vi "Main.vi"   [LabVIEW 2017, in "PrototypePatternDemo.lvclass"]
uses:
  PrototypePatternDemo.lvclass
  ConsoleOut/Print Options.ctl
  BundledShapeCache Class/BundledShapeCache.lvclass
  Shape Class/pShape.lvclass
  Circle Class/pCircle.lvclass
  Rectangle Class/pRectangle.lvclass
  C:/Users/fflores/Documents/LabVIEW-Open-Projects/LabIVEW OOP Design Patterns/Prototype Pattern/Shape Class/pShape.lvclass
types:
  T1 = typedef "Print Options.ctl" = enum16{"Create", "Get Reference", "Print", "Print Header", "Close"}
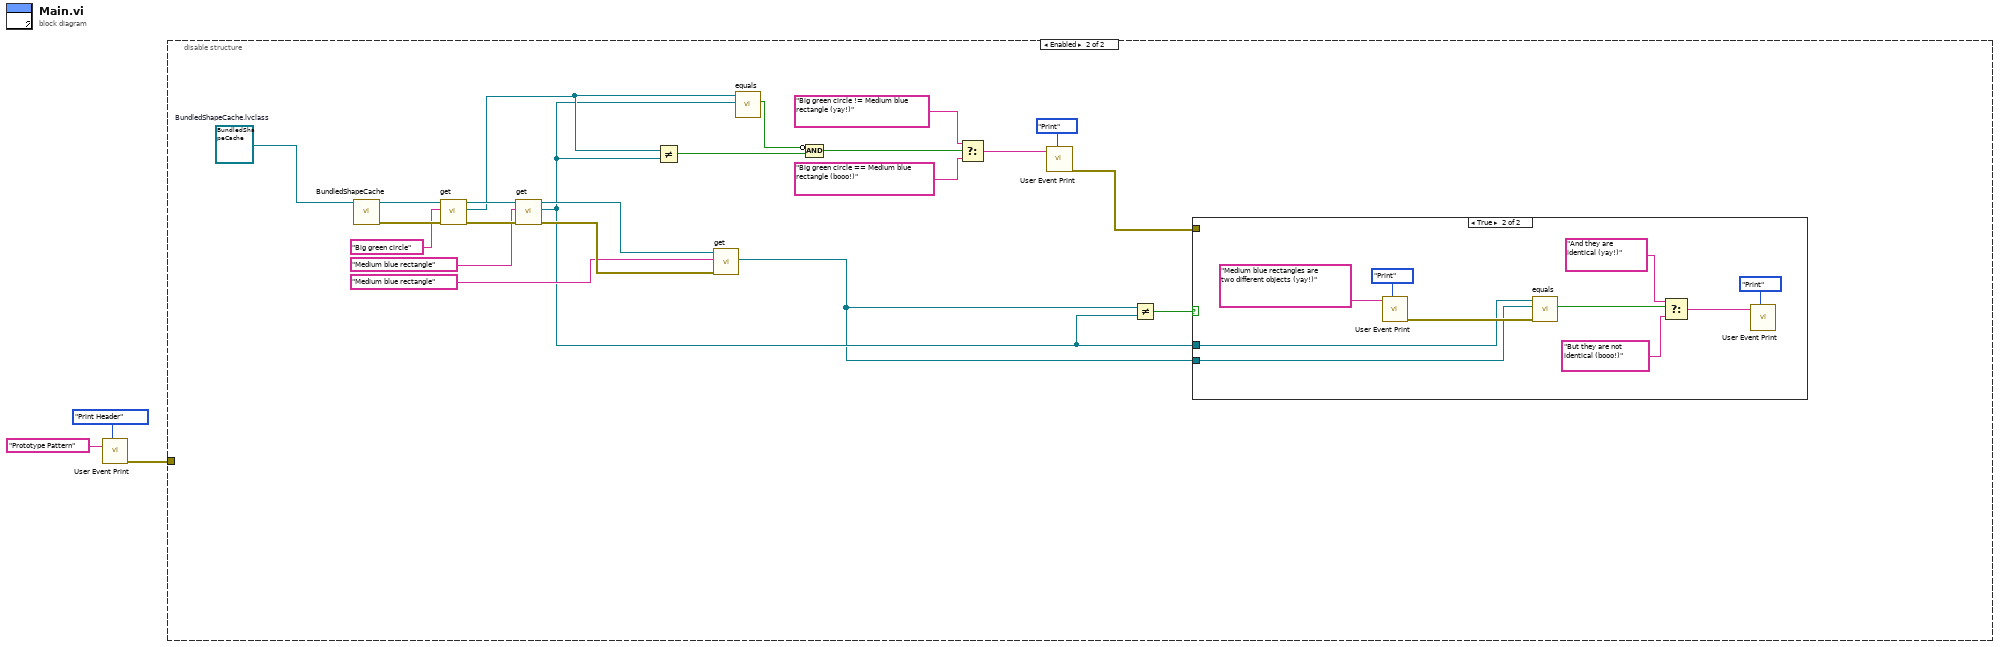
[diagram p0: block diagram]
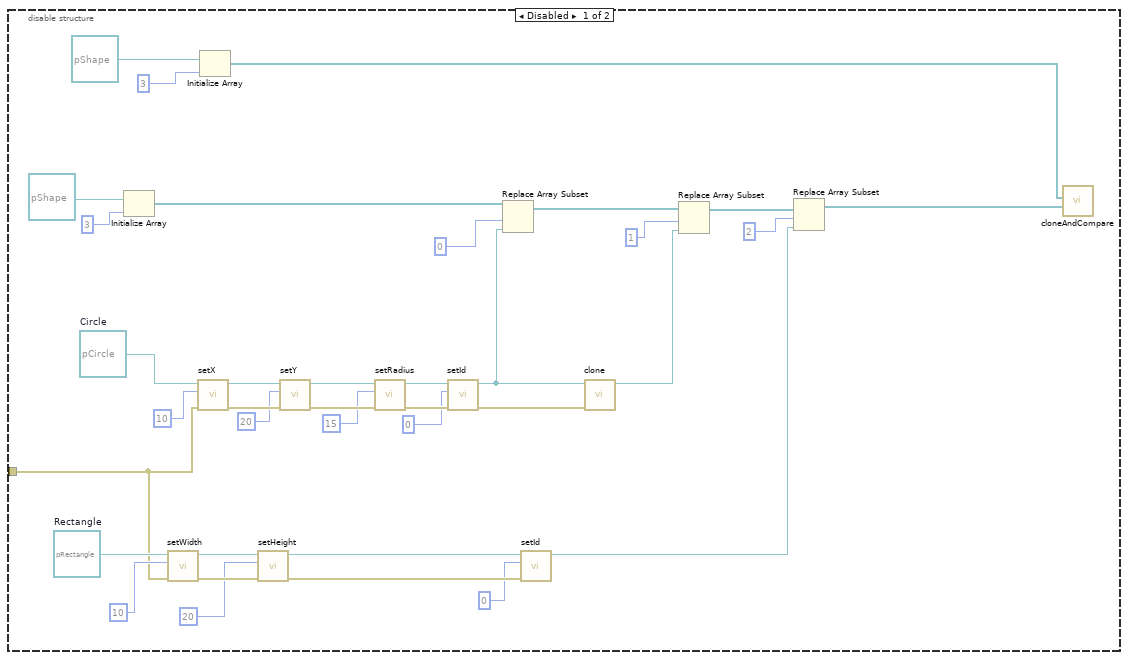
[diagram p2: hidden frame]
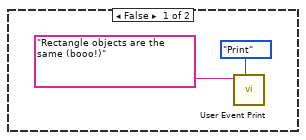
[diagram p3: hidden frame]
diagram:
  n1 = call "User Event Print.vi"("Options"=Print_Options."Print Header", "String to Print"="Prototype Pattern") -> ("error out"=w3:errorcluster)  [unwired: 8 in, 1 out]
  n2 = disable-structure shown="Enabled" {
    disable-tunnel: w3 -> [w12 _]
    frame Disabled {
      w28 = refnum<class "pRectangle.lvclass"> refnum  # Rectangle
      w35 = refnum<class "pCircle.lvclass"> refnum  # Circle
      n3 = Initialize Array(refnum<class "pShape.lvclass"> refnum ("pShape.lvclass"), 3 ("dimension size")) -> (w23:refnum<class "pShape.lvclass">[])
      n4 = call "setWidth.vi"("error in (no error)"=w12, "width"=10, "pRectangle in"=w28) -> ("error out"=w29:errorcluster, "pRectangle out"=w30:refnum<class "pRectangle.lvclass">)  [unwired: 7 in]
      n5 = call "setX.vi"("error in (no error)"=w12, "x"=10, "pCircle in"=w35) -> ("error out"=w38:errorcluster, "pCircle out"=w39:refnum<class "pCircle.lvclass">)  [unwired: 7 in]
      n6 = Initialize Array(refnum<class "pShape.lvclass"> refnum ("pShape.lvclass"), 3 ("dimension size")) -> (w15:refnum<class "pShape.lvclass">[])
      n7 = call "setHeight.vi"("error in (no error)"=w29, "height"=20, "pRectangle in"=w30) -> ("error out"=w5:errorcluster, "pRectangle out"=w21:refnum<class "pRectangle.lvclass">)  [unwired: 7 in]
      n8 = call "setY.vi"("error in (no error)"=w38, "y"=20, "pCircle in"=w39) -> ("error out"=w36:errorcluster, "pCircle out"=w37:refnum<class "pCircle.lvclass">)  [unwired: 7 in]
      n9 = call "setRadius.vi"("error in (no error)"=w36, "radius"=15, "pCircle in"=w37) -> ("error out"=w32:errorcluster, "pCircle out"=w10:refnum<class "pCircle.lvclass">)  [unwired: 7 in]
      n10 = call-dynamic "setId.vi"("error in (no error)"=w32, "ID"=0, "pCircle in"=w10) -> ("error out"=w11:errorcluster, "pCircle out"=w8:refnum<class "pCircle.lvclass">)  [unwired: 7 in]
      n11 = Replace Array Subset "Replace Array Subset"(array=w23, new element=w8, index=0) -> (w31:refnum<class "pShape.lvclass">[])
      n12 = call-dynamic "setId.vi"("error in (no error)"=w5, "ID"=0, "pRectangle in"=w21) -> ("pRectangle out"=w6:refnum<class "pRectangle.lvclass">)  [unwired: 7 in, 1 out]
      n13 = call-dynamic "clone.vi"("error in (no error)"=w11, "pCircle in"=w8) -> ("pCircle out"=w13:refnum<class "pCircle.lvclass">)  [unwired: 8 in, 1 out]
      n14 = Replace Array Subset(array=w31, new element=w13, index=1) -> (w27:refnum<class "pShape.lvclass">[])
      n15 = Replace Array Subset(array=w27, new element=w6, index=2) -> (w14:refnum<class "pShape.lvclass">[])
      n16 = call "cloneAndCompare.vi"("shapes"=w14, "shapesCopy"=w15) -> ()  [unwired: 10 in]
    }
    frame Enabled {
      w61 = refnum<class "BundledShapeCache.lvclass"> refnum  # BundledShapeCache.lvclass
      n17 = call "BundledShapeCache.vi"("BundledShapeCache in"=w61) -> ("error out"=w60:errorcluster, "BundledShapeCache out"=w56:refnum<class "BundledShapeCache.lvclass">)  [unwired: 9 in]
      n18 = call "get.vi"("error in (no error)"=w60, "Key"="Big green circle", "BundledShapeCache in"=w56) -> ("error out"=w58:errorcluster, "pShape.lvclass"=w52:refnum<class "pShape.lvclass">, "BundledShapeCache out"=w59:refnum<class "BundledShapeCache.lvclass">)  [unwired: 6 in]
      n19 = call "get.vi"("error in (no error)"=w58, "Key"="Medium blue rectangle", "BundledShapeCache in"=w59) -> ("error out"=w57:errorcluster, "pShape.lvclass"=w42:refnum<class "pShape.lvclass">, "BundledShapeCache out"=w44:refnum<class "BundledShapeCache.lvclass">)  [unwired: 6 in]
      n20 = Not Equal?(x=w52, y=w42) -> (x != y?=w50:bool)
      n21 = call "get.vi"("error in (no error)"=w57, "Key"="Medium blue rectangle", "BundledShapeCache in"=w44) -> ("pShape.lvclass"=w41:refnum<class "pShape.lvclass">)  [unwired: 6 in, 2 out]
      n22 = call-dynamic "equals.vi"("object 2"=w42, "pShape in"=w52) -> ("equal?"=w51:bool)  [unwired: 7 in, 2 out]
      n23 = Compound Arithmetic op=AND(invert w51, w50) -> (w48:bool)
      n24 = Select(t="Big green circle != Medium blue rectangle (yay!)", s=w48, f="Big green circle == Medium blue rectangle (booo!)") -> (s? t:f=w46:string)
      n25 = call "User Event Print.vi"("Options"=Print_Options."Print", "String to Print"=w46) -> ("error out"=w40:errorcluster)  [unwired: 8 in, 1 out]
      n26 = Not Equal?(x=w41, y=w42) -> (x != y?=w43:bool)
      n27 = case shown="True" w43 {
        tunnel: w42 -> [_ w70]
        tunnel: w41 -> [_ w69]
        tunnel: w40 -> [_ _]
        frame False {
          n28 = call "User Event Print.vi"("Options"=Print_Options."Print", "String to Print"="Rectangle objects are the same (booo!)") -> ()  [unwired: 8 in, 2 out]
        }
        frame True {
          n29 = call "User Event Print.vi"("Options"=Print_Options."Print", "String to Print"="Medium blue rectangles are two different objects (yay!)") -> ("error out"=w71:errorcluster)  [unwired: 8 in, 1 out]
          n30 = call-dynamic "equals.vi"("error in (no error)"=w71, "object 2"=w69, "pShape in"=w70) -> ("equal?"=w66:bool)  [unwired: 6 in, 2 out]
          n31 = Select(t="And they are identical (yay!)", s=w66, f="But they are not identical (booo!)") -> (s? t:f=w67:string)
          n32 = call "User Event Print.vi"("Options"=Print_Options."Print", "String to Print"=w67) -> ()  [unwired: 8 in, 2 out]
        }
      }
    }
  }
